vi "mainObjectivesRegistrationEtl_2.vi"() -> ()   [LabVIEW 2017]
uses:
  getComputerName.vi
  globalDevices.vi
  globalUtilities.vi
  <vilib>/Analysis/NI_AALBase.lvlib
panel:
  out "xy cal i":i32
  out "element 2":dbl
  out "out":dbl[][](array[numeric])
  out "element":dbl
  out "y value 3":dbl
  out "y value 2":dbl
  out "y value":dbl
  out "subarray 2":dbl[][](array[numeric])
  out "subarray":dbl[][](array[numeric])
  out "appended array":dbl[][](array[numeric])
  out "setting etl1 to":dbl
  out "folder name":string
  in  "redgreen":bool
  out "Intensity Graph":u16[][](graph)
  out "XY Graph 6":cluster{"X":dbl, "Y":dbl}[](graph)
  out "XY Graph 5":cluster{"X":dbl, "Y":dbl}[](graph)
  out "XY Graph 4":cluster{"X":dbl, "Y":dbl}[](graph)
  out "XY Graph 3":cluster{"X":dbl, "Y":dbl}[](graph)
  out "XY Graph 2":cluster{"X":dbl, "Y":dbl}[](graph)
  out "XY Graph":cluster{"X":dbl, "Y":dbl}[](graph)
  out "curr etl0 pos (index)":i32
  out "dpt0[dpt1]":dbl[](array[numeric])=[-1.3290463804486958, -1.2316305979268645, -1.1212630461318092, -1.0138414017259925, -0.9077086052642437, -0.7879824961067727, -0.6552620830414349, -0.5431711241489464, -0.4247559983519593, -0.3094500332450975, -0.18905192370600912, -0.06093037048920009, 0.06463589071459266, 0.2196498896905996, 0.3584540083954262, 0.4919160251092355, 0.6311778325996011, 0.7706641387872266, 0.9159712492967972, 1.0737300085708255, 1.2329966463874322]
  in  "etl1 Q-1":i32=20
  out "N^2 +M galvo":i32
  out "curr. etl1 pos (index)":i32
  out "curr. galvo pos (index)":i32
  out "opendisplayvolume":bool=TRUE
  in  "frames per second":dbl=20.0
  in  "etl0 P-1":i32=40
  in  "galvo N-1":i32=3
  # "REGISTRATION BETWEEN GALVO AND CAMERA"
  # "To produce the Red-Green transformation, after running this VI with redgreen=true, use subvi/subvi-gmmreg/gmmregRegisterRedAndGreen."
  # "Acquisition parameters"
  # "# of etl \npositions to scan"
  # "40 20 for normal operation"
  # "sqrt# of galvo positions in grid\n(without symmetry breaking)"
  # "To set the extent of the galvo scan, use globalDevices.vi."
  # "0. No iris closed after tunable lens, lenses released, laser on, camera released."
  # "1. After the ETL scan ends, the Display Volume vi will open. Select a rectangle to locate the\n    two-photon spot.\n2. After the galvo scan ends, the Display VI will open again. Select a point where you want to shine\n    light, to test the registration."
  # "Always check that the [dpt1] values are reasonable. -->\nIf not, rerun the fits and correct, using basic/test/gaussianFitTestWithData"
  # "When this button is on, open the VI (if it hasn't opened yet by itself)\nsubvi/subvi-acquisitionUtilities/acquisitionDisplayVolume.vi"
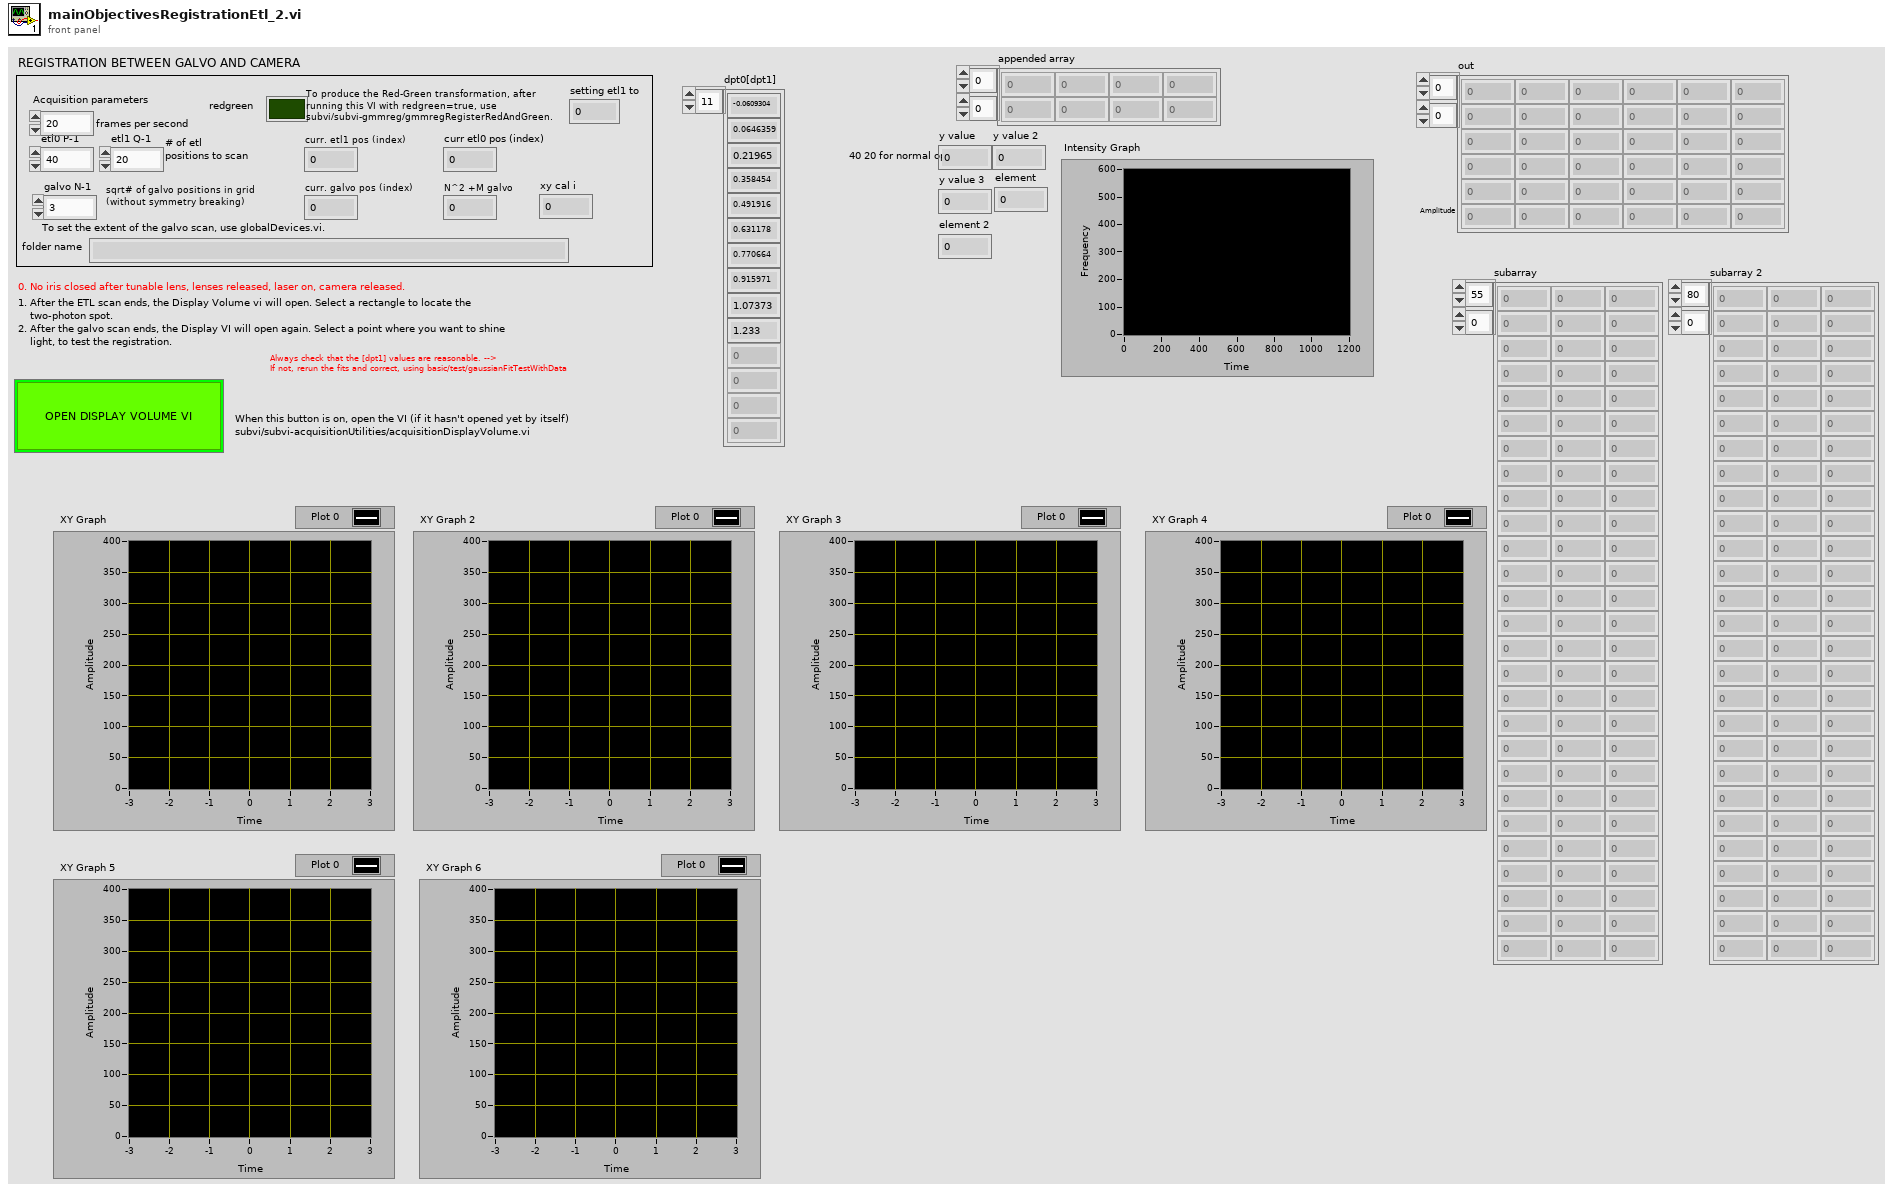
[diagram p1: front panel]
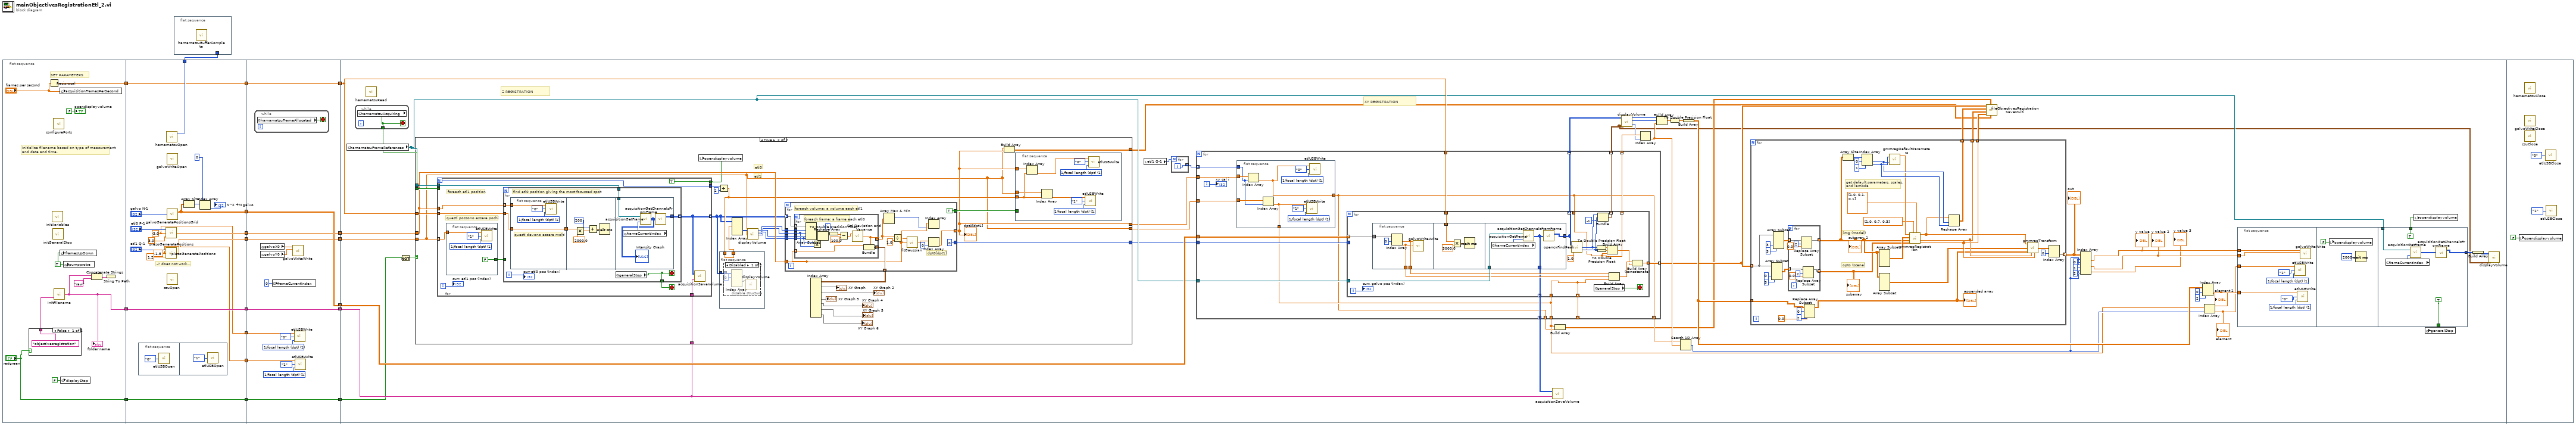
[diagram p0: block diagram]
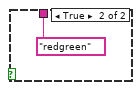
[diagram p2: hidden frame]
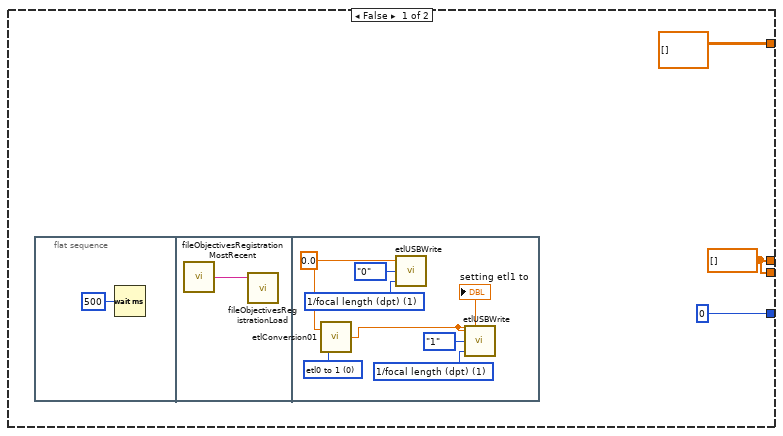
[diagram p3: hidden frame]
diagram:
  n1 = flat-sequence {
    tunnel: [w25] -> w16
    tunnel: [w22] -> w12
    tunnel: ["redgreen"] -> w7
    tunnel: [w46] -> w18
    tunnel: [w37] -> w17
    tunnel: w16 -> [w43]
    tunnel: [w43] -> w15
    tunnel: [w42] -> w14
    tunnel: [w38] -> w13
    tunnel: w12 -> [w38]
    tunnel: [w34] -> w11
    tunnel: [w32] -> w10
    tunnel: [w33] -> w9
    tunnel: [w31] -> w8
    tunnel: w7 -> [w31]
    tunnel: w17 -> [w64]
    tunnel: [w64] -> w6
    tunnel: [w63] -> w5
    tunnel: w15 -> [w63]
    tunnel: [w62] -> w4
    tunnel: w14 -> [w62]
    tunnel: [w61] -> w3
    tunnel: w13 -> [w61]
    tunnel: w11 -> [w60]
    tunnel: [w60] -> w2
    tunnel: w10 -> [w54]
    tunnel: w9 -> [w53]
    tunnel: [w50] -> w1
    tunnel: w8 -> [w50]
    tunnel: w6 -> [w103]
    tunnel: w5 -> [w113]
    tunnel: w4 -> [w115]
    tunnel: w3 -> [w102]
    tunnel: w2 -> [w104]
    tunnel: w1 -> [w101]
    frame #0 {
      w23 = TRUE ("pumpprobe")
      # "SET PARAMETERS"
      # "Initialize filename based on type of measurement\nand date and time."
      n2 = case shown="False" "redgreen" {
        tunnel: ["objectivesregistration" ("Experiment type") "redgreen" ("Experiment type")] -> w21
        frame False {
        }
        frame True {
        }
      }
      n3 = Reciprocal(x="frames per second") -> (1/x=w25:dbl)
      n4 = call "initVariables.vi"() -> ()  [unwired: 12 in]
      n5 = call "initGeneralStop.vi"() -> ()  [unwired: 1 in]
      n6 = call "configurePorts.vi"() -> ()  [unwired: 12 in]
      n7 = call "initFilename.vi"("Experiment type"=w21) -> ("folder name"=w22:string)  [unwired: 1 in]
      "folder name" <- w22
      n8 = global write "globalUtilities.vi" "framesUpDown"(w23) -> ()
      n9 = global write "globalUtilities.vi" "acquisitionFramesPerSecond"("frames per second") -> ()
      n10 = global write "globalUtilities.vi" "displayStop"(FALSE ("displayStop")) -> ()
      n11 = global write "globalUtilities.vi" "pumpprobe"(w23) -> ()
      n12 = Concatenate Strings(w22, "raw") -> (w28:string)
      n13 = String To Path(string=w28) -> ()  [unwired: 1 out]
      "opendisplayvolume" <- FALSE ("OPEN DISPLAY VOLUME")
    }
    frame #1 {
      w33 = -1.5 ("z0")
      w32 = -3.0 ("z0")
      # "-7 does not work..."
      n14 = flat-sequence {
        frame #0 {
          n15 = call "etlUSBOpen.vi"("lens"=enum16{"0", "1"}."0") -> ()  [unwired: 1 in, 1 out]
        }
        frame #1 {
          n16 = call "etlUSBOpen.vi"("lens"=enum16{"0", "1"}."1") -> ()  [unwired: 1 in, 1 out]
        }
      }
      n17 = call "piezoGeneratePositions.vi"("zf"=1.2, "z0"=w33, "M"="etl1 Q-1") -> ("positions (z)"=w34:dbl[])
      n18 = call "piezoGeneratePositions.vi"("zf"=3.0, "z0"=w32, "M"="etl0 P-1") -> ("positions (z)"=w37:dbl[])
      n19 = call "hamamatsuOpen.vi"() -> ("Handle out"=w46:u32)  [unwired: 3 out]
      n20 = call "galvoWriteOpen.vi"() -> ()  [unwired: 12 in]
      n21 = call "galvoGeneratePositionsGrid.vi"("N-1"="galvo N-1") -> ("grid"=w42:dbl[][])  [unwired: 1 out]
      n22 = call "csuOpen.vi"() -> ()  [unwired: 14 in, 2 out]
      n23 = Array Size(array=w42) -> (size(s)=w41:i32[])
      n24 = Index Array(array=w41, index=0) -> (element=→"N^2 +M galvo":i32)
    }
    frame #2 {
      w55 = u16 1 items=["position (um)", "1/focal length (dpt)"] ("mode")
      w58 = u16 1 items=["position (um)", "1/focal length (dpt)"] ("mode")
      n25 = while {
        stop <- w65 stop-if-true
        n26 = global read "globalDevices.vi" "hamamatsuFrameAllocated"() -> (w65:bool)
      }
      n27 = global read "globalDevices.vi" "galvoX0"() -> (w52:dbl)
      n28 = global read "globalDevices.vi" "galvoY0"() -> (w51:dbl)
      n29 = global write "globalUtilities.vi" "frameCurrentIndex"(0 ("frameCurrentIndex")) -> ()
      n30 = call "galvoWriteWrite.vi"("X"=w52, "Y"=w51) -> ()  [unwired: 4 in]
      n31 = call "etlUSBWrite.vi"("mode"=w55, "lens"=enum16{"0", "1"}."0", "input"=w54) -> ()  [unwired: 1 in]
      n32 = call "etlUSBWrite.vi"("mode"=w58, "lens"=enum16{"0", "1"}."1", "input"=w53) -> ()  [unwired: 1 in]
    }
    frame #3 {
      # "XY REGISTRATION"
      # "Z REGISTRATION"
      n33 = global read "globalDevices.vi" "hamamatsuFrameReferences"() -> (w111:refnum<data-value>[])
      n34 = while {
        tunnel: [w348] -> w114
        stop <- w348 stop-if-true
        n35 = global read "globalUtilities.vi" "hamamatsuAcquiring"() -> (w348:bool)
      }
      n36 = call "hamamatsuRead.vi"() -> ()  [unwired: 12 in]
      n37 = Not(x=w101) -> (.not. x?=w100:bool)
      n38 = case shown="True" w100 {
        tunnel: w114 -> [_ w252]
        tunnel: w113 -> [_ w251]
        tunnel: w111 -> [_ w250]
        tunnel: [0 w249] -> w105
        tunnel: [dbl[][] [] w248] -> w72
        tunnel: w104 -> [_ w225]
        tunnel: w103 -> [_ w246]
        tunnel: w102 -> [_ w244]
        tunnel: [w213 w226] -> w98
        tunnel: [w213 w225] -> w99
        frame False {
          w213 = dbl[] []
          n39 = flat-sequence {
            frame #0 {
              n40 = Wait (ms)(milliseconds to wait=u32 500) -> ()  [unwired: 1 out]
            }
            frame #1 {
              n41 = call "fileObjectivesRegistrationMostRecent.vi"() -> ("f"=w217:string)  [unwired: 1 in]
              n42 = call "fileObjectivesRegistrationLoad.vi"("objectiveRegistrationFilePath"=w217) -> ()  [unwired: 3 in, 6 out]
            }
            frame #2 {
              w219 = u16 0 items=["etl0 to 1", "etl1 to 0"] ("mode")
              w220 = 0.0 ("input")
              w224 = u16 1 items=["position (um)", "1/focal length (dpt)"] ("mode")
              w221 = u16 1 items=["position (um)", "1/focal length (dpt)"] ("mode")
              n43 = call "etlConversion01.vi"("mode"=w219, "in"=w220) -> ("out"=w218:dbl)
              "setting etl1 to" <- w218
              n44 = call "etlUSBWrite.vi"("mode"=w224, "lens"=enum16{"0", "1"}."0", "input"=w220) -> ()  [unwired: 1 in]
              n45 = call "etlUSBWrite.vi"("mode"=w221, "lens"=enum16{"0", "1"}."1", "input"=w218) -> ()  [unwired: 1 in]
            }
          }
        }
        frame True {
          # "etl0"
          # "etl1"
          n46 = for {
            N -> [w294]
            tunnel: w250 -> [w295]
            tunnel: w251 -> [w296]
            tunnel: [TRUE] -> w243
            tunnel: w252 -> [_]
            tunnel: [w288] -> w227 mode=indexing
            tunnel: [w294] -> w242
            tunnel: w225 -> [w293] mode=indexing
            tunnel: w246 -> [w292]
            tunnel: w244 -> [w289]
            i -> [w297]
            stop <- w290 stop-if-true
            # "foreach etl1 position"
            # "questi possono essere pochi"
            n47 = flat-sequence {
              tunnel: w293 -> [w322]
              tunnel: [FALSE] -> w291
              frame #0 {
                w320 = u16 1 items=["position (um)", "1/focal length (dpt)"] ("mode")
                n48 = call "etlUSBWrite.vi"("mode"=w320, "lens"=enum16{"0", "1"}."1", "input"=w322) -> ()  [unwired: 1 in]
              }
            }
            n49 = for {
              tunnel: w292 -> [w305] mode=indexing
              tunnel: w296 -> [w303]
              tunnel: w295 -> [w302]
              tunnel: [w301] -> w288 mode=indexing
              tunnel: w291 -> [_]
              tunnel: [w299] -> w290
              i -> [w300]
              stop <- w299 stop-if-true
              # "find etl0 position giving the most focussed spot"
              n50 = flat-sequence {
                tunnel: w305 -> [w307]
                tunnel: [w306] -> w304
                tunnel: w303 -> [w306]
                tunnel: w304 -> [w312]
                tunnel: w302 -> [w317]
                tunnel: [w316] -> w301
                frame #0 {
                  w309 = u16 1 items=["position (um)", "1/focal length (dpt)"] ("mode")
                  # "questi devono essere molti"
                  n51 = call "etlUSBWrite.vi"("mode"=w309, "lens"=enum16{"0", "1"}."0", "input"=w307) -> ()  [unwired: 1 in]
                }
                frame #1 {
                  n52 = Multiply(x=w312, y=2000.0) -> (x*y=w310:dbl)
                  n53 = Add(x=200, y=w310) -> (x+y=w314:dbl)
                  n54 = Wait (ms)(milliseconds to wait=w314) -> ()  [unwired: 1 out]
                }
                frame #2 {
                  n55 = global read "globalUtilities.vi" "frameCurrentIndex"() -> (w318:i32)
                  n56 = call "acquisitionGetFrame.vi"("index"=w318, "hamamatsuFrameReferences"=w317) -> ("frameOut"=w315:u16[][])
                  "Intensity Graph" <- w315
                  n57 = call "acquisitionGetChannelsFromFrame.vi"("frameIn"=w315) -> ("Red"=w316:u16[][])  [unwired: 1 out]
                }
              }
              n58 = global read "globalUtilities.vi" "generalStop"() -> (w299:bool)
              "curr etl0 pos (index)" <- w300
            }
            n59 = call "acquisitionSaveVolume.vi"("folder"=w289, "volume"=w288) -> ()  [unwired: 1 in]
            "curr. etl1 pos (index)" <- w297
          }
          n60 = local write "opendisplayvolume"(w243) -> ()
          n61 = Divide(x=w242, y=2) -> (x/y=w245:dbl)
          n62 = flat-sequence {
            tunnel: w245 -> [w254]
            tunnel: [w254] -> w228
            tunnel: w227 -> [w253]
            frame #0 {
              n63 = disable-structure shown="Disabled" {
                disable-tunnel: w253 -> [w257 _]
                frame Disabled {
                  n64 = Index Array(array=w257, index (dim 0)=0 ("index (vol)")) -> (element=w255:u16[][][])  [unwired: 3 in]
                  n65 = call "displayVolume.vi"("frames"=w255) -> ()  [unwired: 13 in, 6 out]
                }
                frame Enabled {
                }
              }
            }
          }
          n66 = Index Array(array=w227, index (dim 0)=w228) -> (element=w240:u16[][][])  [unwired: 3 in]
          n67 = call "displayVolume.vi"("frames"=w240, "z"=w225) -> ("X0out"=w239:i32, "deltaXout"=w238:i32, "Y0out"=w237:i32, "deltaYout"=w236:i32)  [unwired: 12 in, 2 out]
          n68 = for {
            tunnel: w227 -> [w268] mode=indexing
            tunnel: w239 -> [w273]
            tunnel: w238 -> [w272]
            tunnel: w237 -> [w271]
            tunnel: w236 -> [w270]
            tunnel: [w261] -> w226 mode=indexing
            tunnel: [0] -> w249
            tunnel: w246 -> [w263]
            tunnel: [TRUE] -> w247
            tunnel: [w264] -> w235 mode=indexing
            # "dpt0[dpt1]"
            # "foreach volume; a volume each etl1"
            n69 = for {
              tunnel: w268 -> [w287] mode=indexing
              tunnel: w273 -> [w286]
              tunnel: w272 -> [w282]
              tunnel: w271 -> [w285]
              tunnel: w270 -> [w283]
              tunnel: [w274] -> w260 mode=indexing
              tunnel: w263 -> [w280] mode=indexing
              tunnel: [w279] -> w264 mode=indexing
              # "foreach frame; a frame each etl0"
              n70 = Array Subset(array=w287, index (row)=w285, length (row)=w283, index (col)=w286, length (col)=w282) -> (w284:u16[][])
              n71 = Multiply(x=w282, y=w283) -> (x*y=w281:i32)
              n72 = Reshape Array(w284, w281) -> (w278:u16[])
              n73 = To Double Precision Float(number=w278) -> (double precision float=w277:dbl[])
              n74 = Subtract(x=w277, y=100.0) -> (x-y=w276:dbl[])
              n75 = call <vilib>:"Std Deviation and Variance.vi"("X"=w276) -> ("standard deviation"=w274:dbl)  [unwired: 1 in, 2 out]
              n76 = Bundle(w280, "standard deviation"=w274) -> (w279:cluster{dbl, "standard deviation":dbl})  [unwired: 1 in]
            }
            n77 = Array Max & Min(array=w260) -> (max index (indices)=w262:i32)  [unwired: 3 out]
            n78 = Divide(x=w260, y=1.0) -> (x/y=w259:dbl[])
            n79 = call "fitGaussian.vi"("X"=w263, "Y"=w259) -> ("x0,sigma,bg,amplitude"=w266:dbl[])  [unwired: 1 in]
            n80 = Index Array(array=w263, index=w262) -> ()  [unwired: 1 out]
            n81 = Index Array(array=w266, index=0) -> (element=w261:dbl)
          }
          "dpt0[dpt1]" <- w226
          n82 = Index Array(array=w235) -> (element #1=→"XY Graph":cluster{dbl, "standard deviation":dbl}[], element #2=→"XY Graph 2":cluster{dbl, "standard deviation":dbl}[], element #3=→"XY Graph 3":cluster{dbl, "standard deviation":dbl}[], element #4=→"XY Graph 4":cluster{dbl, "standard deviation":dbl}[], element #5=→"XY Graph 5":cluster{dbl, "standard deviation":dbl}[], element #6=→"XY Graph 6":cluster{dbl, "standard deviation":dbl}[])  [unwired: 12 in]
          n83 = Build Array(w225, w226) -> (w248:dbl[][])
          n84 = flat-sequence {
            tunnel: w226 -> [w326]
            tunnel: w245 -> [w325]
            tunnel: w225 -> [w323]
            tunnel: w247 -> [_]
            frame #0 {
              w329 = u16 1 items=["position (um)", "1/focal length (dpt)"] ("mode")
              w330 = u16 1 items=["position (um)", "1/focal length (dpt)"] ("mode")
              n85 = Index Array(array=w326, index=w325) -> (element=w324:dbl)
              n86 = Index Array(array=w323, index=w325) -> (element=w327:dbl)
              n87 = call "etlUSBWrite.vi"("mode"=w329, "lens"=enum16{"0", "1"}."1", "input"=w327) -> ()  [unwired: 1 in]
              n88 = call "etlUSBWrite.vi"("mode"=w330, "lens"=enum16{"0", "1"}."0", "input"=w324) -> ()  [unwired: 1 in]
            }
          }
        }
      }
      n89 = local read "etl1 Q-1"() -> (w68:i32)
      n90 = for {
        N: w68 -> [_]
        tunnel: [w116] -> w67 mode=indexing
        i -> [w116]
      }
      n91 = for {
        tunnel: w115 -> [w171]
        tunnel: w113 -> [w170]
        tunnel: [w169] -> w90 mode=concatenating
        tunnel: [w168] -> w76 mode=indexing
        tunnel: w111 -> [w167]
        tunnel: [w166] -> w66 mode=indexing
        tunnel: [w165] -> w106 mode=concatenating
        tunnel: w105 -> [w164]
        tunnel: w98 -> [w162]
        tunnel: w99 -> [w163]
        tunnel: w67 -> [w161] mode=indexing
        tunnel: [w160] -> w95 mode=concatenating
        tunnel: [w159] -> _ mode=concatenating
        tunnel: [w157] -> w78 mode=indexing
        tunnel: [w158] -> w71 mode=indexing
        tunnel: [w157] -> w70 mode=indexing
        i -> [w156]
        n92 = flat-sequence {
          tunnel: w162 -> [w176]
          tunnel: w163 -> [w175]
          tunnel: w161 -> [w174]
          tunnel: [w173] -> w157
          tunnel: [w172] -> w158
          frame #0 {
            w178 = u16 1 items=["position (um)", "1/focal length (dpt)"] ("mode")
            w179 = u16 1 items=["position (um)", "1/focal length (dpt)"] ("mode")
            n93 = Index Array(array=w176, index=w174) -> (element=w173:dbl)
            n94 = Index Array(array=w175, index=w174) -> (element=w172:dbl)
            n95 = call "etlUSBWrite.vi"("mode"=w178, "lens"=enum16{"0", "1"}."1", "input"=w172) -> ()  [unwired: 1 in]
            n96 = call "etlUSBWrite.vi"("mode"=w179, "lens"=enum16{"0", "1"}."0", "input"=w173) -> ()  [unwired: 1 in]
          }
        }
        n97 = for {
          tunnel: w171 -> [w201] mode=indexing
          tunnel: w170 -> [w200]
          tunnel: w167 -> [w199]
          tunnel: [w196] -> w169 mode=indexing
          tunnel: [w195] -> w166 mode=indexing
          tunnel: [w189] -> w168 mode=indexing
          tunnel: [w185] -> w165 mode=indexing
          tunnel: w164 -> [_]
          tunnel: w157 -> [w182]
          tunnel: w158 -> [w181]
          tunnel: [w182] -> w160 mode=indexing
          tunnel: [w181] -> w159 mode=indexing
          i -> [w197]
          stop <- w184 stop-if-true
          n98 = flat-sequence {
            tunnel: w201 -> [w205]
            tunnel: [w203] -> w192
            tunnel: [w202] -> w191
            tunnel: w200 -> [w207]
            tunnel: w199 -> [w211]
            tunnel: [w210] -> w196
            tunnel: [w209] -> w185
            frame #0 {
              n99 = Index Array(array=w205, index #1=0 ("index")) -> (element #1=w203:dbl, element #2=w202:dbl)  [unwired: 1 in]
              n100 = call "galvoWriteWrite.vi"("X"=w203, "Y"=w202) -> ()  [unwired: 4 in]
            }
            frame #1 {
              n101 = Multiply(x=w207, y=3000.0) -> (x*y=w206:dbl)
              n102 = Wait (ms)(milliseconds to wait=w206) -> ()  [unwired: 1 out]
            }
            frame #2 {
              n103 = global read "globalUtilities.vi" "frameCurrentIndex"() -> (w212:i32)
              n104 = call "acquisitionGetFrame.vi"("index"=w212, "hamamatsuFrameReferences"=w211) -> ("frameOut"=w209:u16[][])
              n105 = call "acquisitionGetChannelsFromFrame.vi"("frameIn"=w209) -> ("Red"=w210:u16[][])  [unwired: 1 out]
            }
          }
          n106 = call "opencvFindPeak.vi"("blur"=1.0, "Image (2D)"=w196) -> ("maxLocY"=w187:i32, "maxLocX"=w188:i32)
          n107 = global read "globalUtilities.vi" "generalStop"() -> (w184:bool)
          n108 = To Double Precision Float(number=w188) -> (double precision float=w194:dbl)
          n109 = To Double Precision Float(number=w187) -> (double precision float=w193:dbl)
          n110 = Bundle("maxLocX"=w188, "maxLocY"=w187, -1) -> (w195:cluster{"maxLocX":i32, "maxLocY":i32, i32})  [unwired: 1 in]
          n111 = Build Array(w194, w193, w182) -> (w186:dbl[])
          n112 = Build Array(w192, w191, w181) -> (w190:dbl[])
          n113 = Build Array (concatenate)(w190, w186) -> (w189:dbl[])
          "curr. galvo pos (index)" <- w197
        }
        "xy cal i" <- w156
      }
      n114 = call "acquisitionSaveVolume.vi"("folder"=w102, "volume"=w106) -> ()  [unwired: 1 in]
      n115 = Build Array(w71, w70) -> (w69:dbl[][])
      n116 = call "displayVolume.vi"("frames"=w90, "overlay (z:-1 all planes)"=w66) -> ("X0out"=w112:i32, "Y0out"=w94:i32, "zout (plane index)"=w83:i32)  [unwired: 12 in, 3 out]
      n117 = Index Array(array=w95, index=w83) -> (element=w79:dbl)
      n118 = Build Array(w112, w94, w79) -> (w97:dbl[])
      n119 = To Double Precision Float(number=w97) -> (double precision float=w96:dbl[])
      n120 = Search 1D Array(1D array=w78, element=w79) -> (index of element=w77:i32)  [unwired: 1 in]
      n121 = Build Array(w96) -> (w93:dbl[][])
      n122 = for {
        tunnel: [w147] -> w73 mode=indexing
        tunnel: w76 -> [w136] mode=indexing
        tunnel: [w134] -> w74 mode=indexing
        tunnel: [w133] -> w75 mode=indexing
        tunnel: w93 -> [w119]
        tunnel: [w126] -> w89 mode=indexing
        # "get default parameters, scales,\nand lambda"
        # "img (model)"
        # "opto (scene)"
        n123 = Array Subset(array=w136, index (col)=0 ("index"), length (col)=3 ("length")) -> (w123:dbl[][])  [unwired: 2 in]
        n124 = Array Subset(array=w136, index (col)=3 ("index"), length (col)=3 ("length")) -> (w125:dbl[][])  [unwired: 2 in]
        n125 = for {
          tunnel: w125 -> [w155] mode=indexing
          tunnel: [w152] -> w124 mode=indexing
          tunnel: w123 -> [w149] mode=indexing
          tunnel: [w148] -> w122 mode=indexing
          n126 = Replace Array Subset(array=w155, new element=0.0 ("new element/subarray"), index=2) -> (w152:dbl[])
          n127 = Replace Array Subset(array=w149, new element=0.0 ("new element/subarray"), index=2) -> (w148:dbl[])
        }
        "subarray" <- w122
        "subarray 2" <- w124
        n128 = Replace Array Subset(array=w119, new element=0.0 ("new element/subarray"), index (row)=0 ("index"), index (col)=2 ("disabled index (col)")) -> (w117:dbl[][])
        "appended array" <- w117
        n129 = Array Size(array=w124) -> (size(s)=w143:i32[])
        n130 = Index Array(array=w143, index #1=0 ("index"), index #2=1 ("index")) -> (element #1=w145:i32, element #2=w146:i32)
        n131 = Array Subset(array=w124) -> (w131:dbl[][])  [unwired: 4 in]
        n132 = Array Subset(array=w124) -> (w132:dbl[][])  [unwired: 4 in]
        n133 = call "gmmregDefaultParameters.vi"("D (3)"=w146, "nctrlPts"=w145) -> ("param0"=w144:dbl[])  [unwired: 3 out]
        n134 = call "gmmregRegistration.vi"("lambda"=dbl[] [1.0, 0.1, 0.1], "scale"=dbl[] [1.0, 0.7, 0.3], "scene"=w122, "model"=w124, "ctrlPoints"=w132, "param0"=w144) -> ("denormParams out"=w133:dbl[], "normParams out"=w134:dbl[], "param0 out"=w135:dbl[])  [unwired: 2 in, 1 out]
        n135 = Reshape Array(w135, w145, w146) -> (w147:dbl[][])
        n136 = call "gmmregTransform.vi"("param0"=w135, "ctrlPts"=w131, "pts"=w117, "normParams"=w134, "denormParams"=w133) -> ("out"=w128:dbl[][])  [unwired: 4 in]
        n137 = Index Array(array=w128, index (row)=0) -> (element=w126:dbl[])  [unwired: 1 in]
      }
      "out" <- w89
      n138 = call "fileObjectivesRegistrationSaveMulti.vi"("z(opto)z(img)"=w72, "z(opto,img) of xy registrations"=w69, "denormParam"=w75, "normParam"=w74, "param"=w73, "xyz(opto)xyz(img)"=w76) -> ()  [unwired: 1 in]
      n139 = Index Array(array=w89, index (row) #1=w77, index (col) #1=0 ("disabled index (col)"), index (row) #2=w77, index (col) #2=1 ("index (col)"), index (row) #3=w77, index (col) #3=2 ("index (col)")) -> (element #1=w82:dbl, element #2=w81:dbl, element #3=→"y value 3":dbl)
      "y value" <- w82
      "y value 2" <- w81
      n140 = Index Array(array=w93, index (row)=0, index (col)=2 ("disabled index (col)")) -> (element=w85:dbl)
      "element 2" <- w85
      n141 = Index Array(array=w71, index=w77) -> (element=w84:dbl)
      "element" <- w84
      n142 = flat-sequence {
        tunnel: w82 -> [w339]
        tunnel: w81 -> [w338]
        tunnel: w84 -> [w333]
        tunnel: w85 -> [w332]
        tunnel: w111 -> [w346]
        tunnel: [w342] -> w110
        tunnel: [TRUE] -> w108
        tunnel: [TRUE ("opendisplayvolume")] -> w107
        frame #0 {
          w335 = u16 1 items=["position (um)", "1/focal length (dpt)"] ("mode")
          w336 = u16 1 items=["position (um)", "1/focal length (dpt)"] ("mode")
          n143 = call "etlUSBWrite.vi"("mode"=w336, "lens"=enum16{"0", "1"}."1", "input"=w333) -> ()  [unwired: 1 in]
          n144 = call "etlUSBWrite.vi"("mode"=w335, "lens"=enum16{"0", "1"}."0", "input"=w332) -> ()  [unwired: 1 in]
          n145 = call "galvoWriteWrite.vi"("X"=w339, "Y"=w338) -> ()  [unwired: 4 in]
        }
        frame #1 {
          n146 = local write "opendisplayvolume"(FALSE ("opendisplayvolume")) -> ()
          n147 = Wait (ms)(milliseconds to wait=u32 2000) -> ()  [unwired: 1 out]
        }
        frame #2 {
          n148 = global read "globalUtilities.vi" "frameCurrentIndex"() -> (w347:i32)
          n149 = call "acquisitionGetFrame.vi"("index"=w347, "hamamatsuFrameReferences"=w346) -> ("frameOut"=w343:u16[][])
          n150 = call "acquisitionGetChannelsFromFrame.vi"("frameIn"=w343) -> ("Red"=w342:u16[][])  [unwired: 1 out]
        }
      }
      n151 = local write "opendisplayvolume"(w107) -> ()
      n152 = global write "globalUtilities.vi" "generalStop"(w108) -> ()
      n153 = Build Array(w110) -> (w109:u16[][][])
      n154 = call "displayVolume.vi"("frames"=w109, "overlay (z:-1 all planes)"=w66) -> ()  [unwired: 12 in, 6 out]
    }
    frame #4 {
      n155 = local write "opendisplayvolume"(FALSE ("opendisplayvolume")) -> ()
      n156 = call "hamamatsuClose.vi"() -> ()  [unwired: 1 out]
      n157 = call "galvoWriteClose.vi"() -> ()  [unwired: 12 in]
      n158 = call "csuClose.vi"() -> ()  [unwired: 12 in]
      n159 = call "etlUSBClose.vi"("lens"=enum16{"0", "1"}."0") -> ()  [unwired: 1 in]
      n160 = call "etlUSBClose.vi"("lens"=enum16{"0", "1"}."1") -> ()  [unwired: 1 in]
    }
  }
  n161 = flat-sequence {
    tunnel: w18 -> [_]
    frame #0 {
      n162 = call "hamamatsuBufferComplete.vi"() -> ()  [unwired: 12 in]
    }
  }
